vi "timer.vi"(10 "Time":dbl, 11 "In":bool) -> (3 "Out":bool)   [LabVIEW 2012]
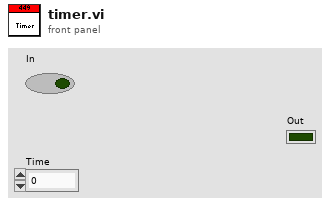
[diagram p1: front panel]
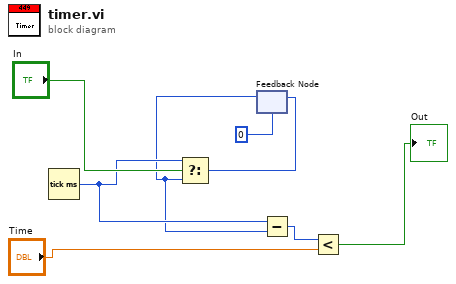
[diagram p0: block diagram]
diagram:
  n1 = Tick Count (ms)() -> (millisecond timer value=w6:u32)
  n2 = feedback #1(u32 0 ("millisecond timer value")) -> (w5:u32)
  n3 = Select(t=w6, s="In", f=w5) -> (s? t:f=w7:u32)
  n4 = feedback-in #1(w7) -> ()
  n5 = Subtract(x=w6, y=w5) -> (x-y=w4:u32)
  n6 = Less?(x=w4, y="Time") -> (x < y?=→"Out":bool)
